vi "LowPass.vi"(6 "filter":fxp<+/-,16,1>=0.100006103515625, 10 "DAC in":fxp<+/-,20,5>) -> (2 "DAC out":fxp<+/-,20,5>)   [LabVIEW 2014]
doc: "low pass time constant is 1/filter samples, 1 = no filter, 0.1 = 10 sample time constant. Inputs and outputs 20,5 fixed point for 16-bit DACs."
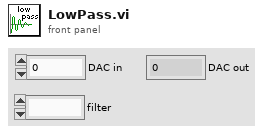
[diagram p1: front panel]
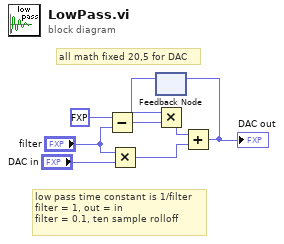
[diagram p0: block diagram]
diagram:
  # "all math fixed 20,5 for DAC"
  # "low pass time constant is 1/filter\nfilter = 1, out = in\nfilter = 0.1, ten sample rolloff"
  n1 = Subtract(x=fxp<+/-,20,5> 1.0 ("filter"), y="filter") -> (x-y=w8:fxp<+/-,20,5>)
  n2 = Multiply(x="filter", y="DAC in") -> (x*y=w6:fxp<+/-,20,5>)
  n3 = feedback #1() -> (w2:fxp<+/-,20,5>)  [unwired: 1 in]
  n4 = Multiply(x=w2, y=w8) -> (x*y=w7:fxp<+/-,40,10>)
  n5 = Add(x=w7, y=w6) -> (x+y=w1:fxp<+/-,20,5>)
  "DAC out" <- w1
  n6 = feedback-in #1(w1) -> ()
